vi "MES_Delete Parmeters.vi"(0 "Main":string="0", 1 "Name":string="0", 2 "CMD":T1(ring)=enum."Read", 5 "VariableName":string, 9 "Value":string, 11 "error in (no error)":errorcluster, 12 "GiveAlarm?":bool=TRUE) -> (15 "error out":errorcluster)   [LabVIEW 2021, in "SQLite.lvclass"]
doc: "更新Parameter表格里面的Value和Unit，根据输入的不同而更新不同的内容。\n2015-06-25 23:34:20\n蒋松\njiangsong@outlook.com"
uses:
  SQLite.lvclass
  SQLiteFileName.ctl
  TabelFullName.ctl
  <vilib>/Utility/error.llb/Trim Whitespace.vi
  SQLite.lvclass/SQLite.ctl
  <userlib>/sushu/sushu.lvlib
  <userlib>/LabSQL/LabSQL.lvlib
panel:
  out "Select SQL CMD":string
  out "concatenated string":string
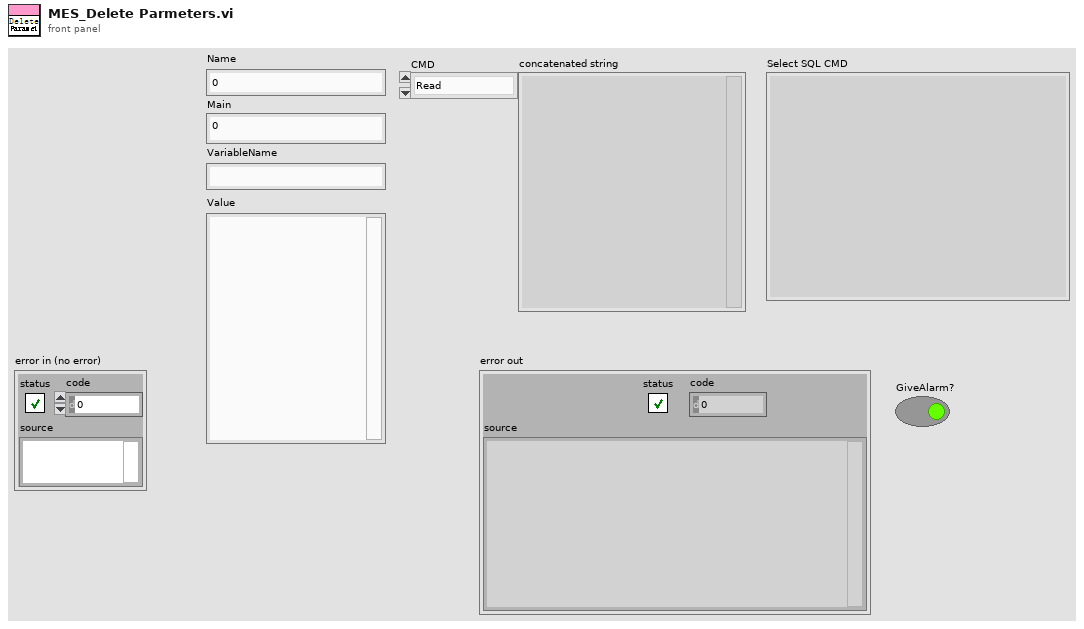
[diagram p1: front panel]
types:
  T1 = enum16{"Initialize", "Read", "Write", "UnInitialize"}
  T2 = typedef "SQLite.lvclass/TabelFullName.ctl" = string
  T3 = typedef "SQLite.lvclass/SQLiteFileName.ctl" = string
  T4 = cluster{"Current VI Reference":refnum<vi>, "Close Panel on Exit?":bool}
  T5 = cluster{"Core":cluster{"Current VI Reference":refnum<vi>, "Close Panel on Exit?":bool}, "VI Name":string}
  T6 = enum32{"invalid app kind", "Development System", "Run Time System", "Student Edition", "Embedded LabVIEW", "Evaluation", "Custom"}
  T7 = enum32{"Invalid", "Standard", "Closed", "Hidden", "Minimized", "Maximized"}
  T8 = enum16{"Other", "SQL2008", "SQLite", "Access", "MySQL"}
  T9 = enum16{"String", "Long (I32)", "Single (SGL)", "Double (DBL)", "Date/Time", "Binary"}[]
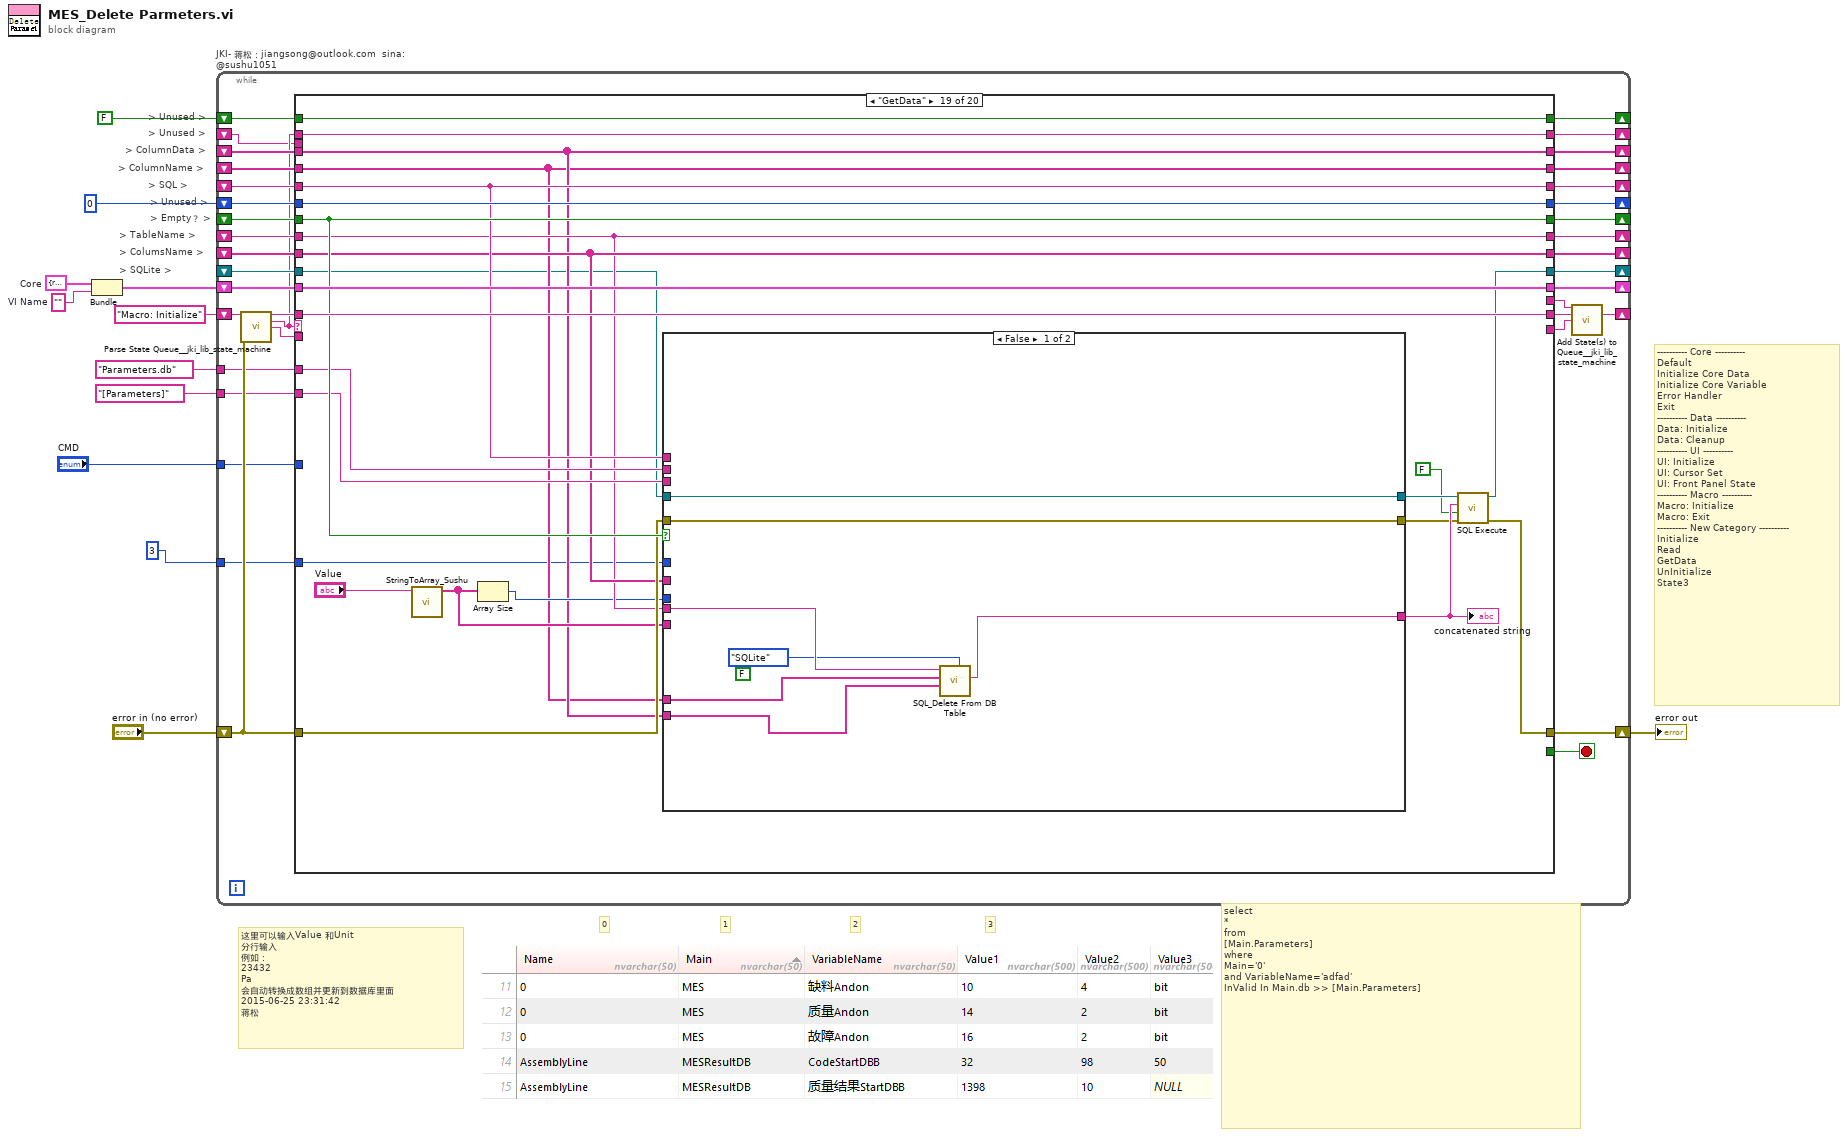
[diagram p0: block diagram]
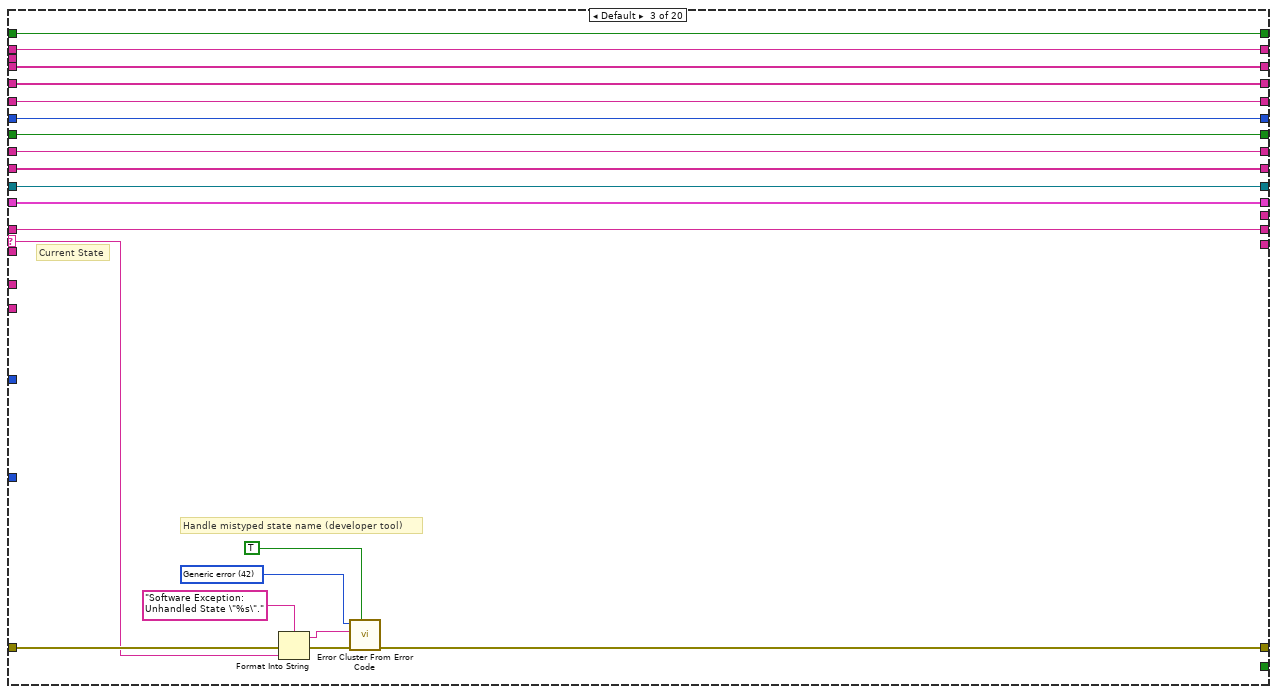
[diagram p4: hidden frame]
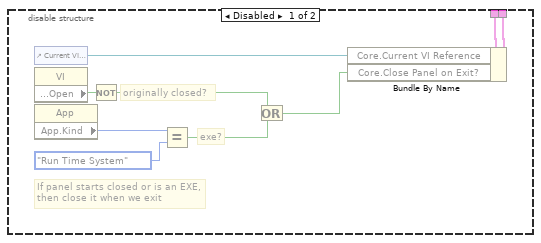
[diagram p6: hidden frame]
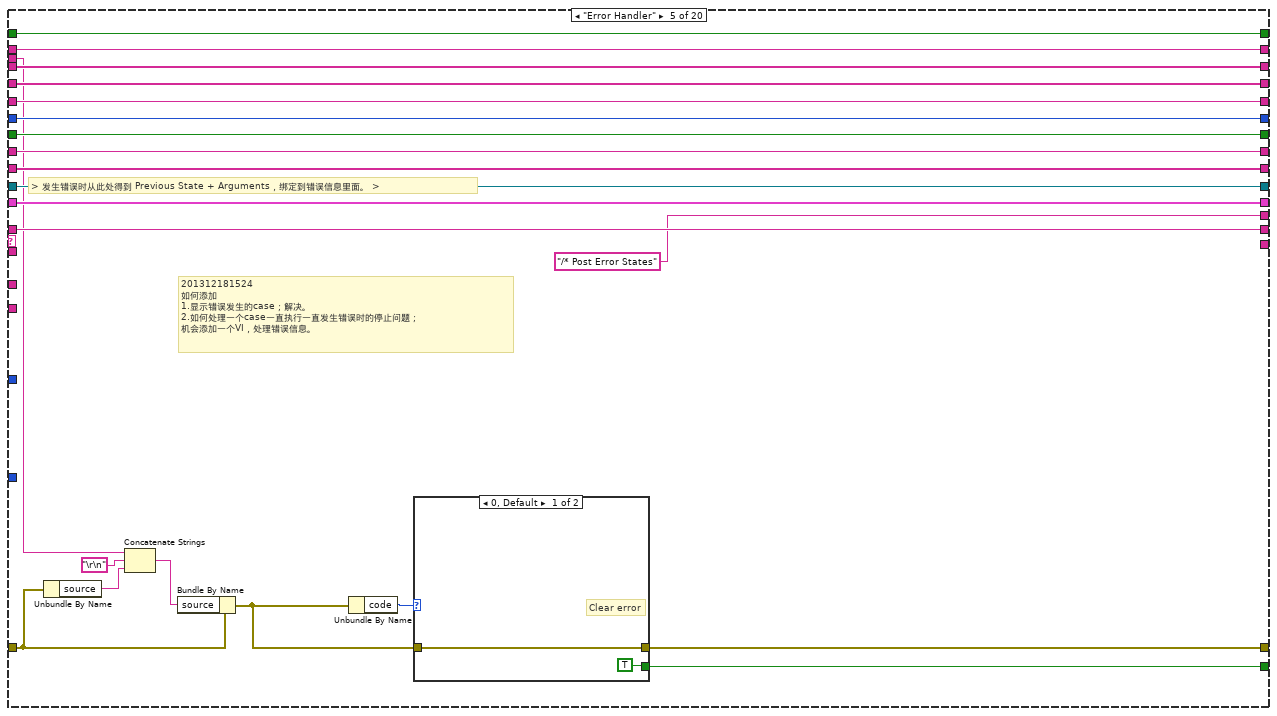
[diagram p7: hidden frame]
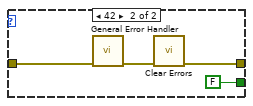
[diagram p8: hidden frame]
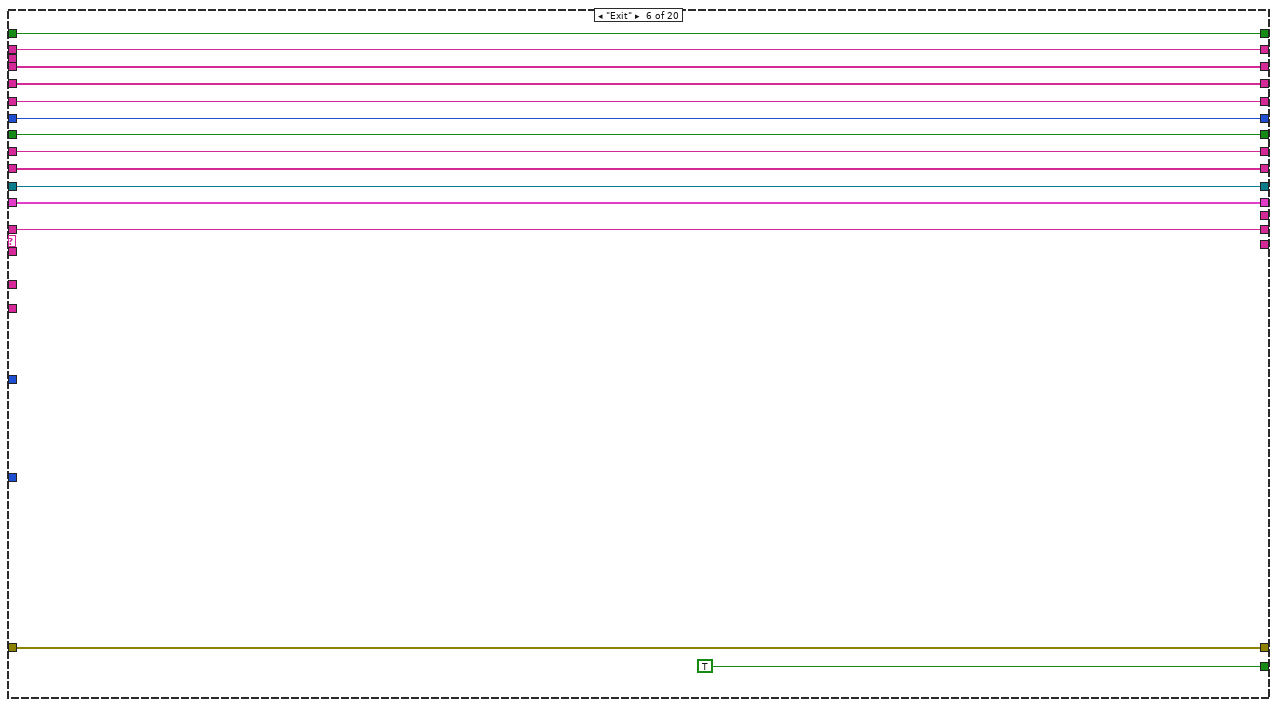
[diagram p9: hidden frame]
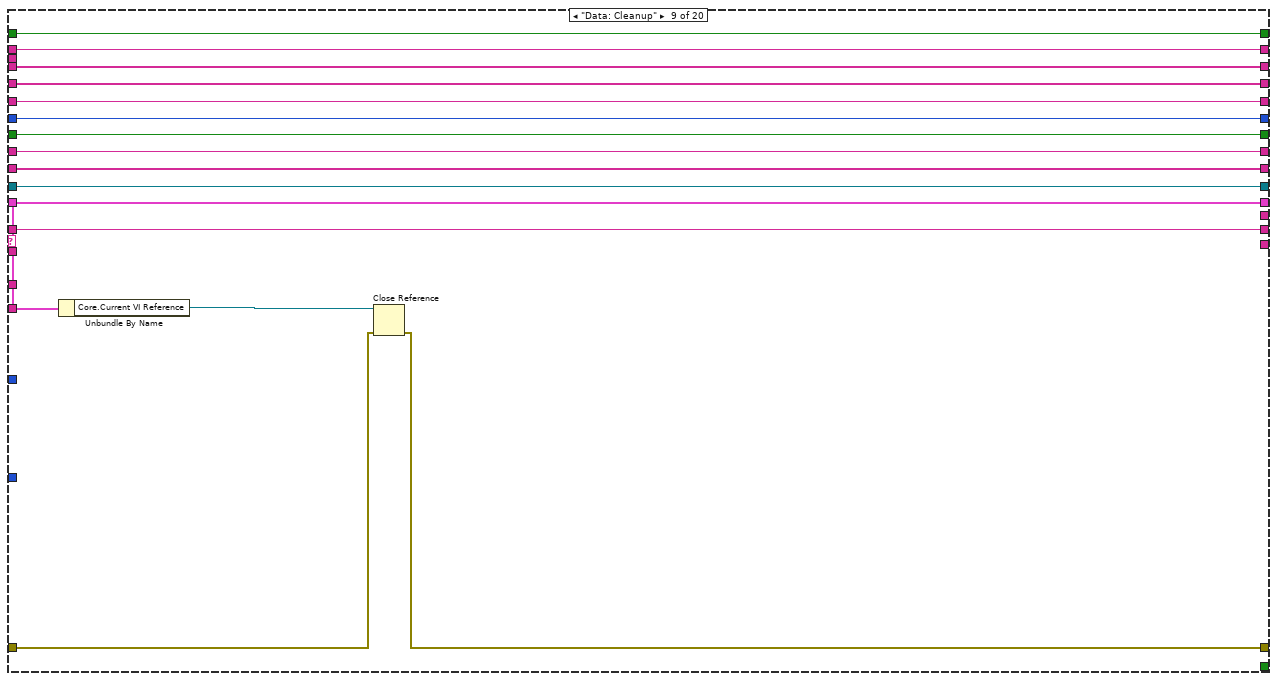
[diagram p12: hidden frame]
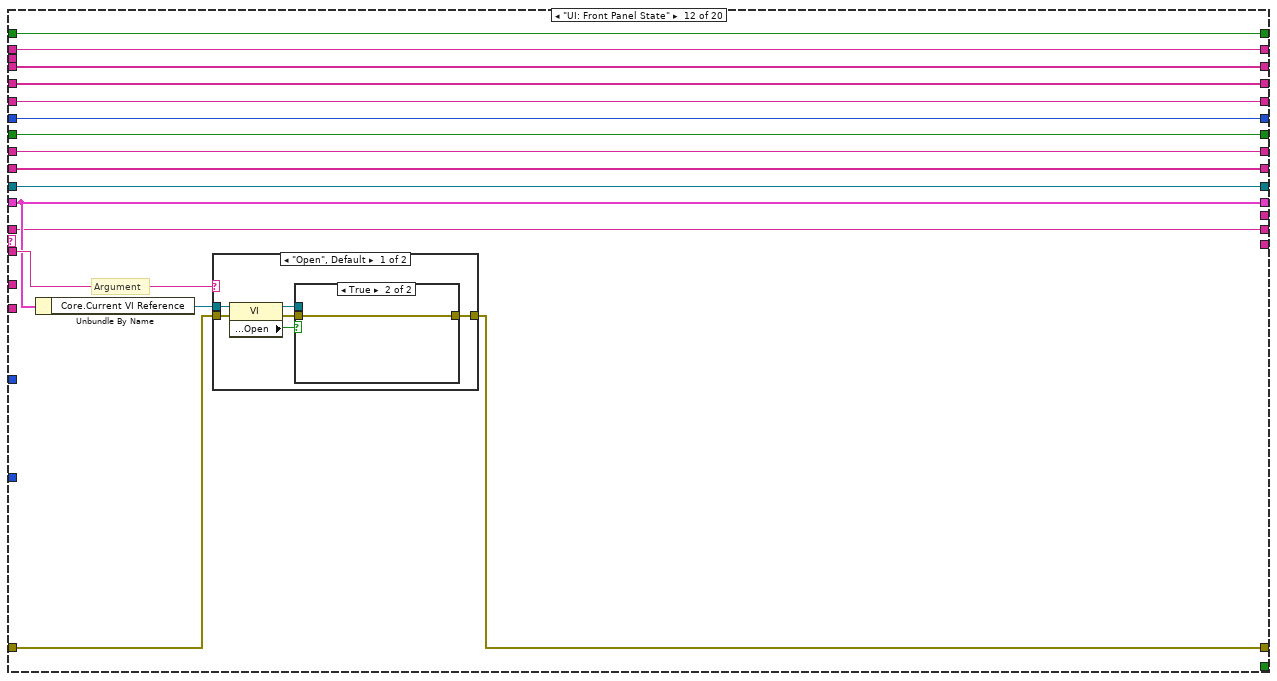
[diagram p15: hidden frame]
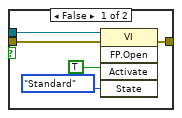
[diagram p16: hidden frame]
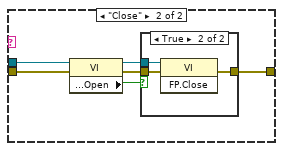
[diagram p17: hidden frame]
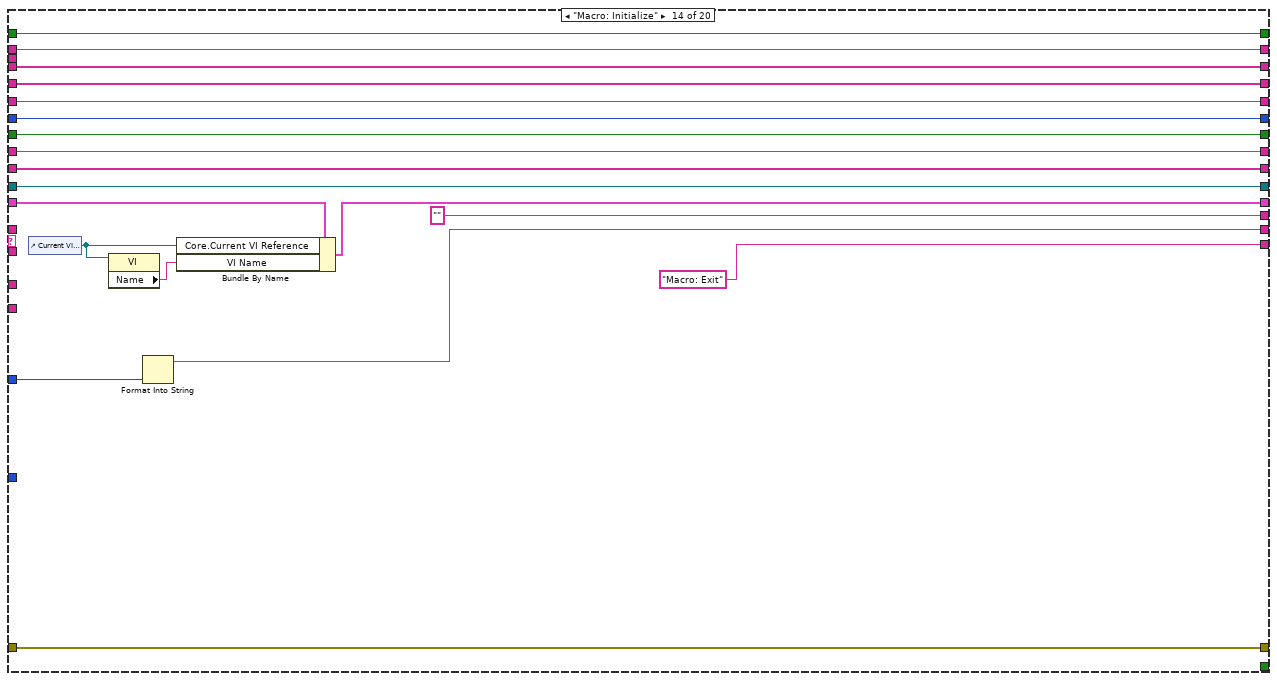
[diagram p20: hidden frame]
diagram:
  w12 = ""  # VI Name
  w11 = T4 {"Current VI Reference"=refnum, "Close Panel on Exit?"=FALSE}  # Core
  # "> Unused >"
  # "> SQL >"
  # "> ColumnName >"
  # "> ColumnData >"
  # "> Unused >"
  # "> Unused >"
  # "> SQLite >"
  # "> ColumsName >"
  # "> TableName >"
  # "> Empty？ >"
  # "---------- Core ----------\nDefault\nInitialize Core Data\nInitialize Core Variable\nError Handler\nExit\n---------- Data ----------\nData: Initialize\nData: Cleanup\n---------- UI ----------\nUI: Initialize\nUI: Cursor Set\nUI: Front Panel State\n---------- Macro ----------\nMacro: Initialize\nMacro: Exit\n---------- New Category ----------\nInitialize\nRead\nGetData\nUnInitialize\nState3"
  # "3"
  # "2"
  # "1"
  # "0"
  # "select\n*\nfrom\n[Main.Parameters]\nwhere\nMain='0'\nand VariableName='adfad'\nInValid In Main.db >> [Main.Parameters]"
  # "这里可以输入Value 和Unit\n分行输入\n例如：\n23432\nPa\n会自动转换成数组并更新到数据库里面\n2015-06-25 23:31:42\n蒋松"
  n1 = Bundle("Core"=w11, "VI Name"=w12) -> (w10:T5)  [unwired: 1 in]
  n2 = while "JKI- 蒋松：jiangsong@outlook.com  sina: @sushu1051" {
    shift-right: [w47] -> w4
    shift-left: "error in (no error)" -> [w45]
    shift-right: [w34] -> _
    shift-left: "Macro: Initialize" -> [w35]
    shift-right: [w41] -> _
    shift-left: _ -> [w43]
    shift-right: [w42] -> _
    shift-left: _ -> [w44]
    shift-right: [w36] -> _
    shift-left: w10 -> [w39]
    shift-right: [w37] -> _
    shift-left: _ -> [w30]
    shift-right: [w38] -> _
    shift-left: _ -> [w40]
    shift-right: [w29] -> _
    shift-left: 0 -> [w28]
    shift-right: [w21] -> _
    shift-left: _ -> [w19]
    shift-right: [w20] -> _
    shift-left: _ -> [w14]
    shift-right: [w24] -> _
    shift-left: _ -> [w25]
    shift-right: [w23] -> _
    shift-left: _ -> [w22]
    shift-right: [w26] -> _
    shift-left: FALSE -> [w27]
    tunnel: "CMD" -> [w18]
    tunnel: T3 "Parameters.db" ("SQLiteFileName") -> [w17]
    tunnel: T2 "[Parameters]" ("TabelFullName") -> [w16]
    tunnel: 3 ("index") -> [w13]
    stop <- w46 stop-if-true
    n3 = call <vilib>:"Parse State Queue__jki_lib_state_machine.vi"("State Queue"=w35, "Error In (no error)"=w45) -> ("Remaining States"=w49:string, "Current State"=w15:string, "Arguments"=w48:string)  [unwired: 10 in, 1 out]
    n4 = case shown="\"GetData\"" w15 {
      selector: w15 -> [_ _ w83 _ _ _ _ _ _ _ _ _ _ _ _ _ _ w373 _ _]
      tunnel: w49 -> [w62 w69 w82 w102 w133 w154 w168 w182 w194 w209 w222 w235 w273 _ w306 w323 w354 w381 w418 w446]
      tunnel: w48 -> [_ _ _ _ _ _ _ _ _ _ _ w238 _ _ _ _ _ _ _ _]
      tunnel: [w61 w75 w84 w106 w127 w156 w170 w184 w196 w211 w224 w239 w275 w295 w313 w326 w335 w359 w396 w433] -> w47
      tunnel: w45 -> [w61 w75 w85 w106 w137 w156 w170 w184 w197 w211 w224 w240 w275 w295 w313 w326 w340 w361 w412 w432]
      tunnel: [w62 w69 w82 w102 w133 w154 w168 w182 w194 w209 w222 w235 w273 w281 w306 w323 w354 w381 w418 w446] -> w33
      tunnel: [_ _ _ _ w126 TRUE _ _ _ _ _ _ _ _ _ _ _ _ _ _] -> w46
      tunnel: w44 -> [w60 w74 w95 w109 w141 w161 w174 w187 w202 w215 w228 w244 w279 w298 w316 w329 w353 _ w413 w445]
      tunnel: w43 -> [w59 w73 w94 w108 w140 w160 w173 w186 w201 w214 w227 w243 w278 w297 w315 w328 _ w369 w407 w444]
      tunnel: [w60 w74 w95 w109 w141 w161 w174 w187 w202 w215 w228 w244 w279 w298 w316 w329 w353 w368 w413 w445] -> w42
      tunnel: [w59 w73 w94 w108 w140 w160 w173 w186 w201 w214 w227 w243 w278 w297 w315 w328 w336 w369 w407 w444] -> w41
      tunnel: w40 -> [w58 w72 w93 w107 w139 w159 w172 w185 w200 w213 w226 w242 w277 w296 w314 w327 _ w370 w408 w443]
      tunnel: w30 -> [w56 w70 w92 w103 w131 w155 w169 w183 w195 w210 w223 w236 w274 w294 w307 w324 _ w365 w401 w435]
      tunnel: w39 -> [w57 w71 w91 w105 w138 w158 w171 w175 w198 w212 w225 w237 w276 w283 w308 w325 w352 w380 w417 w442]
      tunnel: [w58 w72 w93 w107 w139 w159 w172 w185 w200 w213 w226 w242 w277 w296 w314 w327 w338 w370 w408 w443] -> w38
      tunnel: [w56 w70 w92 w103 w131 w155 w169 w183 w195 w210 w223 w236 w274 w294 w307 w324 w337 w364 w399 w434] -> w37
      tunnel: [w57 w71 w91 w104 w138 w158 w171 w175 w198 w212 w225 w237 w276 w282 w308 w325 w352 w380 w417 w442] -> w36
      tunnel: [_ _ _ _ "/* Post Error States" _ _ _ _ _ _ _ _ "" w305 _ _ w375 _ _] -> w32
      tunnel: [_ _ _ _ _ _ _ _ _ _ _ _ _ "Macro: Exit" _ _ _ _ _ _] -> w31
      tunnel: w28 -> [w55 w68 w81 w101 w130 w153 w167 w181 w193 w208 w221 w234 w272 w293 w304 w322 w351 w376 w416 w441]
      tunnel: [w55 w68 w81 w101 w130 w153 w167 w181 w193 w208 w221 w234 w272 w293 w304 w322 w351 w377 w416 w441] -> w29
      tunnel: w15 -> [w53 w66 w79 w99 w124 w151 w165 w179 w191 w206 w219 w232 w270 w289 w302 w320 w346 w378 w415 w440]
      tunnel: w19 -> [w52 w65 w78 w98 w123 w150 w164 w178 w190 w205 w218 w231 w269 w288 w301 w319 w347 _ w403 w439]
      tunnel: [w53 w66 w79 w99 w124 w151 w165 w179 w191 w206 w219 w232 w270 w289 w302 w320 w346 w378 w415 w440] -> w20
      tunnel: [w52 w65 w78 w98 w123 w150 w164 w178 w190 w205 w218 w231 w269 w288 w301 w319 w347 w366 w403 w439] -> w21
      tunnel: w22 -> [w51 w64 w77 w97 w122 w149 w163 w177 w189 w204 w217 w230 w268 w287 w300 w318 w348 _ w402 w438]
      tunnel: w25 -> [w50 w63 w76 w96 w121 w148 w162 w176 w188 w203 w216 w229 w267 w286 w299 w317 w349 _ w411 w437]
      tunnel: [w51 w64 w77 w97 w122 w149 w163 w177 w189 w204 w217 w230 w268 w287 w300 w318 w348 w367 w402 w438] -> w23
      tunnel: [w50 w63 w76 w96 w121 w148 w162 w176 w188 w203 w216 w229 w267 w286 w299 w317 w349 w363 w411 w437] -> w24
      tunnel: w27 -> [w54 w67 w80 w100 w125 w152 w166 w180 w192 w207 w220 w233 w271 w290 w303 w321 w350 w379 w414 w436]
      tunnel: [w54 w67 w80 w100 w125 w152 w166 w180 w192 w207 w220 w233 w271 w290 w303 w321 w350 w379 w414 w436] -> w26
      tunnel: w18 -> [_ _ _ _ _ _ _ _ _ _ _ _ _ w280 _ _ _ _ _ _]
      tunnel: w17 -> [_ _ _ _ _ _ _ _ _ _ _ _ _ _ _ _ _ _ w410 _]
      tunnel: w16 -> [_ _ _ _ _ _ _ _ _ _ _ _ _ _ _ _ w339 _ w409 _]
      tunnel: w14 -> [_ _ _ _ w120 _ _ _ _ _ _ _ _ _ _ _ _ _ _ _]
      tunnel: w13 -> [_ _ _ _ _ _ _ _ _ _ _ _ _ _ _ _ _ w355 w394 _]
      frame "Idle" {
      }
      frame "---------- Core ----------" {
      }
      frame Default {
        w87 = 42 items=["No error", "Argument error", "Memory is full", "Out of zone", "End of file", "File already open", "Generic file I/O error", "File not found", "File permission error", "Disk is full", "Duplicate path", "Too many files open", "System feature not enabled", "Resource file not found", "Cannot add resource", "Resource not found", "Image not found", "Image memory error", "Pen does not exist", "Config type invalid", "Config token not found", "Config parse error", "Config memory error", "Bad external code format", "Bad external code offset", "External code not present", "Null window", "Destroy window error", "Null menu", "Print aborted", "Bad print record", "Print driver error", "Windows error during printing", "Memory error during printing", "Print dialog error", "Generic print error", "Invalid device refnum", "Device not found", "Device parameter error", "Device unit error", "Cannot open device", "Device call aborted", "Generic error", "Cancelled by user", "Object ID too low", "Object ID too high", "Object not in heap", "Unknown heap", "Unknown object (invalid DefProc)", "Unknown object (DefProc not in table)", "Message out of range", "Invalid (null) method", "Unknown message", "Manager call not supported", "Bad address", "Network operation in progress", "Network operation timed out", "Connection is busy", "Network attribute not supported", "Network error", "Address in use", "System out of memory", "Connection aborted", "Connection refused", "Not connected", "Already connected", "Connection closed", "Initialization error (interapplication manager)", "Bad occurrence", "Wait on unbound occurrence handler", "Occurrence queue overflow", "Datalog type conflict", "Unused", "Unrecognized type (interapplication manager)", "Memory corrupt", "Failed to make temporary DLL", "Old CIN version", "Drag socket not found", "Failed to load drop-object", "Failed to register OLE object", "Failed to release OLE object", "Format specifier type mismatch", "Unknown format specifier", "Too few format specifiers", "Too many format specifiers", "Scan failed", "Newer CIN version", "Error converting to variant", "Runtime menu error", "Password tampered", "Variant attribute not found", "Incompatible variant data type", "Event data is not available", "Event Store is not present", "Occurrence is not found", "Event Queue is not created", "Event info is not available", "Refnum passed is NULL", "Error retrieving Class GUID", "Error retrieving CoClass GUID", "Error retrieving TypeLib GUID.", "Bad built application magic bytes.", "Specific driver is different from the specific driver associated with the Logical Name.", "There is no session opened to the class driver.", "Max Error", "MAX - Error with config objects", "MAX - Error loading configuration", "MAX - Group not supported"]
        # "Current State"
        # "Handle mistyped state name (developer tool)"
        n5 = Format Into String(format string="Software Exception: Unhandled State \"%s\"." ("message"), error in=w85, w83) -> (resulting string=w88:string, error out=w89:errorcluster)  [unwired: 1 in]
        n6 = call <vilib>:"Error Cluster From Error Code.vi"("show call chain? (False)"=TRUE, "error in (no error)"=w89, "error message (\"\")"=w88, "error code (0)"=w87) -> ("error out"=w84:errorcluster)  [unwired: 5 in]
      }
      frame "Initialize Core Data" {
        n7 = disable-structure shown="Enabled" {
          disable-tunnel: w105 -> [w111 w119]
          disable-tunnel: [w110 w119] -> w104
          frame Disabled {
            # "originally closed?"
            # "exe?"
            # "If panel starts closed or is an EXE, then close it when we exit"
            n8 = control-ref of="Current VI Reference"() -> (w118:refnum<vi>)
            n9 = property class="VI"() -> ("Front Panel.Open"=w112:bool)  [unwired: 2 in, 2 out]
            n10 = property class="App"() -> ("App.Kind"=w113:T6)  [unwired: 2 in, 2 out]
            n11 = Not(x=w112) -> (.not. x?=w115:bool)
            n12 = Equal?(x=w113, y=T6."Run Time System" ("Application:Kind")) -> (x = y?=w116:bool)
            n13 = Or(x=w115, y=w116) -> (x .or. y?=w117:bool)
            n14 = Bundle By Name(cluster=w111, "Core.Current VI Reference"=w118, "Core.Close Panel on Exit?"=w117) -> (w110:T5)
          }
          frame Enabled {
          }
        }
      }
      frame "Error Handler" {
        # "> 发生错误时从此处得到 Previous State + Arguments，绑定到错误信息里面。 >"
        # "201312181524\n如何添加\n1.显示错误发生的case；解决。\n2.如何处理一个case一直执行一直发生错误时的停止问题；\n机会添加一个VI，处理错误信息。"
        # "Clear error"
        n15 = Unbundle By Name(w137) -> ("source"=w135:string)
        n16 = Concatenate Strings(w120, "\r\n", w135) -> (w134:string)
        n17 = Bundle By Name(cluster=w137, "source"=w134) -> (w128:errorcluster)
        n18 = Unbundle By Name(w128) -> ("code"=w129:i32)
        n19 = case shown="0, Default" w129 {
          tunnel: [TRUE FALSE] -> w126
          tunnel: w128 -> [w143 w146]
          tunnel: [w143 w144] -> w127
          frame 0, Default {
          }
          frame 42 {
            n20 = call <vilib>:"General Error Handler.vi"("error in (no error)"=w146) -> ("error out"=w145:errorcluster)  [unwired: 10 in, 4 out]
            n21 = call <vilib>:"Clear Errors.vi"("error in (no error)"=w145) -> ("error out"=w144:errorcluster)  [unwired: 5 in, 1 out]
          }
        }
      }
      frame "Exit" {
      }
      frame "---------- Data ----------" {
      }
      frame "Data: Initialize" {
      }
      frame "Data: Cleanup" {
        n22 = Unbundle By Name(w198) -> ("Core.Current VI Reference"=w199:refnum<vi>)
        n23 = Close Reference(reference=w199, error in (no error)=w197) -> (error out=w196:errorcluster)
      }
      frame "---------- UI ----------" {
      }
      frame "UI: Initialize" {
      }
      frame "UI: Front Panel State" {
        # "Argument"
        n24 = Unbundle By Name(w237) -> ("Core.Current VI Reference"=w241:refnum<vi>)
        n25 = case shown="\"Open\", Default" w238 {
          tunnel: w240 -> [w248 w261]
          tunnel: [w250 w262] -> w239
          tunnel: w241 -> [w249 w259]
          frame "Open", Default {
            n26 = property class="VI"(reference=w249, error in=w248) -> (reference out=w246:refnum<vi>, error out=w247:errorcluster, "Front Panel.Open"=w245:bool)
            n27 = case shown="True" w245 {
              tunnel: [w253 w256] -> w250
              tunnel: w247 -> [w252 w256]
              tunnel: w246 -> [w251 _]
              frame False {
                n28 = invoke class="VI" method="FP.Open"(reference=w251, error in=w252, "Activate"=TRUE, "State"=T7."Standard") -> (error out=w253:errorcluster)  [unwired: 1 in, 4 out]
              }
              frame True {
              }
            }
          }
          frame "Close" {
            n29 = property class="VI"(reference=w259, error in=w261) -> (reference out=w258:refnum<vi>, error out=w260:errorcluster, "Front Panel.Open"=w257:bool)
            n30 = case shown="True" w257 {
              tunnel: [w263 w266] -> w262
              tunnel: w260 -> [w263 w265]
              tunnel: w258 -> [_ w264]
              frame False {
              }
              frame True {
                n31 = invoke class="VI" method="FP.Close"(reference=w264, error in=w265) -> (error out=w266:errorcluster)  [unwired: 1 in, 2 out]
              }
            }
          }
        }
      }
      frame "---------- Macro ----------" {
      }
      frame "Macro: Initialize" {
        n32 = control-ref of="Current VI Reference"() -> (w284:refnum<vi>)
        n33 = property class="VI"(reference=w284) -> ("Name"=w285:string)  [unwired: 1 in, 2 out]
        n34 = Format Into String(w280) -> (resulting string=w281:string)  [unwired: 3 in, 1 out]
        n35 = Bundle By Name(cluster=w283, "Core.Current VI Reference"=w284, "VI Name"=w285) -> (w282:T5)
      }
      frame "Macro: Exit" {
        n36 = Unbundle By Name(w308) -> ("Core.Close Panel on Exit?"=w309:bool)
        n37 = Select(t="UI: Front Panel State >> Close", s=w309, f="") -> ()  [unwired: 1 out]
        n38 = call <vilib>:"Add State(s) to Queue__jki_lib_state_machine.vi"("State(s) at Back (\"\")"="Data: Cleanup\nExit") -> ("States Out"=w305:string)  [unwired: 14 in]
      }
      frame "---------- New Category ----------" {
      }
      frame "Initialize" {
        n39 = Concatenate Strings(w339) -> (w336:string)
        n40 = call "Get Main.Parmeters.vi"("Main"="MES", "VariableName"="CurrentMESSQLiteDB" ("Main")) -> ("Value"=w332:string)  [unwired: 6 in, 7 out]
        n41 = Type Cast(type=T3 "Parameters.db" ("SQLiteFileName"), x=w332) -> ()  [unwired: 1 out]
        n42 = call "SQLite File Path.vi"("SQLiteFileName"=T3 "SystemConfig.db" ("*(type *) &x"), "SQLite in"=refnum<class "SQLite.lvclass"> refnum ("SQLite.lvclass")) -> ("string"=w343:string, "SQLite out"=w345:refnum<class "SQLite.lvclass">)  [unwired: 7 in, 1 out]
        n43 = call-dynamic "Open Connection.vi"("error in (no error)"=w340, "ConnectionString"=w343, "HostDB in"=w345) -> ("error out"=w342:errorcluster, "HostDB out"=w341:refnum<class "SQLite.lvclass">)  [unwired: 7 in]
        n44 = call-dynamic "Get Table Columns Name.vi"("error in (no error)"=w342, "TableName"=w336, "HostDB in"=w341) -> ("error out"=w335:errorcluster, "Table_ColunmsList"=w338:string[], "HostDB out"=w337:refnum<class "SQLite.lvclass">)  [unwired: 4 in, 2 out]
      }
      frame "Read" {
        w358 = T9 [] items=["String", "Long (I32)", "Single (SGL)", "Double (DBL)", "Date/Time", "Binary"] ("DB Data Type")
        n45 = Build Array("Name", "Main", "VariableName") -> (w366:string[])
        n46 = Array Subset(array=w370, length=w355) -> (w367:string[])  [unwired: 1 in]
        n47 = call <userlib>:"SQL_Select From DB Table.vi"("DB Data Type"=w358, "DB Type"=T8."SQLite", "ColumnsValue"=w366, "ColumnsNameList"=w367, "TableName"=w369) -> ("Select SQL CMD"=w363:string)  [unwired: 6 in]
        "Select SQL CMD" <- w363
        n48 = call-dynamic "SQL Execute.vi"("error in (no error)"=w361, "Command Text"=w363, "HostDB in"=w365) -> ("error out"=w360:errorcluster, "Table Control"=w362:string[][], "HostDB out"=w364:refnum<class "SQLite.lvclass">)  [unwired: 4 in, 2 out]
        n49 = Empty Array?(array=w362) -> (empty?=w368:bool)
        n50 = case shown="Error" w360 {
          tunnel: w360 -> [_ w393]
          tunnel: w376 -> [_ w386]
          tunnel: [w382 w392] -> w375
          tunnel: "GetData" ("f") -> [w382 w391]
          tunnel: w373 -> [_ w388]
          frame No Error {
          }
          frame Error {
            n51 = Unbundle By Name(w393) -> ("status"=w387:bool)
            n52 = Equal?(x=w386, y=0) -> (x = y?=w383:bool)
            n53 = And(x=w387, y=w383) -> (x .and. y?=w384:bool)
            n54 = call <vilib>:"Add State(s) to Queue__jki_lib_state_machine.vi"("State(s) in Front (\"\")"="Initialize" ("Remaining States"), "State(s) in (\"\")"=w388) -> ("States Out"=w389:string)  [unwired: 13 in]
            n55 = Select(t=w389, s=w384, f=w391) -> (s? t:f=w392:string)
          }
        }
        n56 = call <vilib>:"Clear Errors.vi"("error in (no error)"=w360) -> ("error out"=w359:errorcluster)  [unwired: 5 in, 1 out]
        n57 = Increment(x=w376) -> (x+1=w377:i32)
      }
      frame "GetData" {
        n58 = call <userlib>:"StringToArray_Sushu.vi"("State Queue"="Value") -> ("Array"=w404:string[])  [unwired: 7 in, 3 out]
        n59 = Array Size(array=w404) -> (size(s)=w405:i32)
        n60 = case shown="False" w413 {
          tunnel: [w424 w431] -> w397
          tunnel: [w425 w427] -> w400
          tunnel: w404 -> [_ w428]
          tunnel: w408 -> [_ _]
          tunnel: w405 -> [_ _]
          tunnel: w407 -> [w423 _]
          tunnel: w403 -> [w421 w429]
          tunnel: w402 -> [w422 _]
          tunnel: w401 -> [w425 w427]
          tunnel: w412 -> [w424 w431]
          tunnel: w411 -> [_ _]
          tunnel: w410 -> [_ _]
          tunnel: w409 -> [_ _]
          tunnel: [w420 "" ("Insert DB String")] -> w398
          tunnel: w394 -> [_ _]
          frame False {
            (unwired) FALSE ("Check ASCII?")
            n61 = call <userlib>:"SQL_Delete From DB Table.vi"("DB Type"=T8."SQLite", "ColumnsValue"=w421, "ColumnsNameList"=w422, "TableName"=w423) -> ("Select SQL CMD"=w420:string)  [unwired: 7 in]
          }
          frame True {
            # "空，SQL不报错。\n2015-11-03 09:58:24\n蒋松"
            # "变量不存在，自动Insert。\n2015-11-03 09:56:45"
            # "Value处可以多行输入，故要根据Value的数组大小进行相应的索引。\n2015-11-03 09:58:00\n蒋松"
            # "变量不存在，询问是否Insert。\n2015-11-03 09:57:10"
            n62 = Build Array (concatenate)(w429, w428) -> ()  [unwired: 1 out]
            n63 = Not(x="GiveAlarm?") -> ()  [unwired: 1 out]
          }
        }
        "concatenated string" <- w398
        n64 = call-dynamic "SQL Execute.vi"("error in (no error)"=w397, "Return Data (T)"=FALSE, "Command Text"=w398, "HostDB in"=w400) -> ("error out"=w396:errorcluster, "HostDB out"=w399:refnum<class "SQLite.lvclass">)  [unwired: 3 in, 3 out]
      }
      frame "UnInitialize" {
        n65 = call-dynamic "Close Connection.vi"("error in (no error)"=w432, "HostDB in"=w435) -> ("error out"=w433:errorcluster, "HostDB out"=w434:refnum<class "SQLite.lvclass">)  [unwired: 8 in]
      }
    }
    n66 = call <vilib>:"Add State(s) to Queue__jki_lib_state_machine.vi"("State(s) in Front (\"\")"=w32, "State(s) in (\"\")"=w33, "State(s) at Back (\"\")"=w31) -> ("States Out"=w34:string)  [unwired: 12 in]
  }
  "error out" <- w4
